vi "UTIL Predict Class.vi"(4 "Cluster Data From File":dbl[][](array[numeric]), 5 "Data Point":dbl[](array[numeric])) -> (1 "Class":i32)   [LabVIEW 2010]
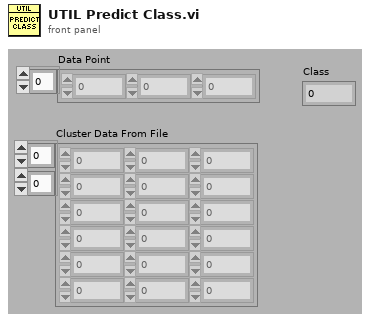
[diagram p1: front panel]
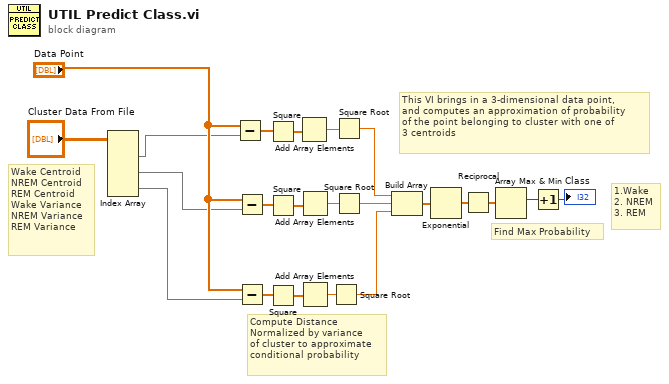
[diagram p0: block diagram]
diagram:
  # "Wake Centroid\nNREM Centroid\nREM Centroid\nWake Variance\nNREM Variance\nREM Variance"
  # "This VI brings in a 3-dimensional data point,\nand computes an approximation of probability\nof the point belonging to cluster with one of \n3 centroids"
  # "1.Wake\n2. NREM\n3. REM"
  # "Find Max Probability"
  # "Compute Distance\nNormalized by variance \nof cluster to approximate \nconditional probability"
  n1 = Index Array(array="Cluster Data From File") -> (element #1=w10:dbl[], element #2=w8:dbl[], element #3=w7:dbl[])  [unwired: 6 in]
  n2 = Subtract(x="Data Point", y=w10) -> (x-y=w4:dbl[])
  n3 = Subtract(x="Data Point", y=w8) -> (x-y=w5:dbl[])
  n4 = Subtract(x="Data Point", y=w7) -> (x-y=w6:dbl[])
  n5 = Square(x=w4) -> (x^2=w1:dbl[])
  n6 = Square(x=w5) -> (x^2=w3:dbl[])
  n7 = Square(x=w6) -> (x^2=w2:dbl[])
  n8 = Add Array Elements(numeric array=w1) -> (sum=w16:dbl)
  n9 = Add Array Elements(numeric array=w3) -> (sum=w17:dbl)
  n10 = Add Array Elements(numeric array=w2) -> (sum=w18:dbl)
  n11 = Square Root(x=w18) -> (sqrt(x)=w21:dbl)
  n12 = Square Root(x=w16) -> (sqrt(x)=w20:dbl)
  n13 = Square Root(x=w17) -> (sqrt(x)=w19:dbl)
  n14 = Build Array(w20, w19, w21) -> (w14:dbl[])
  n15 = Exponential(1:w14) -> (0:w13:dbl[])
  n16 = Reciprocal(x=w13) -> (1/x=w12:dbl[])
  n17 = Array Max & Min(array=w12) -> (max index (indices)=w11:i32)  [unwired: 3 out]
  n18 = Increment(x=w11) -> (x+1=→"Class":i32)
